vi "Get COMM Address.vi"(8 "error in (no error)":errorcluster, 11 "Hardware in":refnum<class "Hardware.lvclass">) -> (0 "error out":errorcluster, 2 "COMM Address":string, 3 "Hardware out":refnum<class "Hardware.lvclass">)   [LabVIEW 2016, in "Hardware.lvlib" / "Hardware.lvclass"]
uses:
  <userlib>/Common Components/Hardware/Abstract Hardware/Hardware.lvclass
  <userlib>/Common Components/Hardware/Abstract Hardware/Hardware.lvclass/Hardware.ctl
  <userlib>/Common Components/Hardware/DevInfo/DevInfo.lvclass/DevInfo.ctl
  <userlib>/Common Components/Hardware/Abstract Hardware/Read DevInfo.vi
  <userlib>/Common Components/Hardware/DevInfo/Read COMM Address.vi
  <userlib>/Common Components/Hardware/DevInfo/DevInfo.lvclass
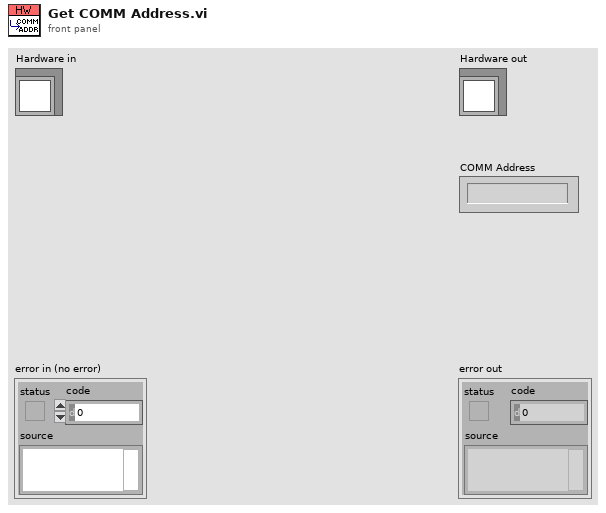
[diagram p1: front panel]
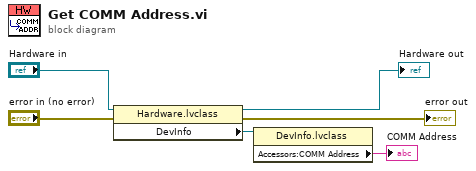
[diagram p0: block diagram]
diagram:
  n1 = property class="Hardware.lvclass"(reference="Hardware in", error in="error in (no error)") -> (reference out=→"Hardware out":refnum<class "Hardware.lvclass">, error out=→"error out":errorcluster, "DevInfo"=w2:refnum<class "DevInfo.lvclass">)
  n2 = property class="DevInfo.lvclass"(reference=w2) -> ("Accessors:COMM Address"=→"COMM Address":string)  [unwired: 1 in, 2 out]
